vi "event_key_down.vi"(8 "error in":errorcluster, 9 "reference cluster in":T1, 11 "Char":i16) -> (0 "error out":errorcluster)   [LabVIEW 2016]
uses:
  Type Definitions/reference_cluster.ctl
  Type Definitions/vars_settings.ctl
  Type Definitions/stim_type.ctl
  Type Definitions/backlight_type.ctl
  Type Definitions/vars_runtime.ctl
  Type Definitions/data.ctl
  Type Definitions/notifier_elements_GUI.ctl
  Type Definitions/notifier_elements_DAQ.ctl
  Type Definitions/notifier_elements_write.ctl
  Type Definitions/control_references.ctl
types:
  T1 = typedef "reference_cluster.ctl" = cluster{"Vars":cluster{"General":refnum<notifier>, "Runtime":refnum<notifier>}, "Data":cluster{"Display":refnum<queue>, "Write":refnum<queue>}, "LoopCtrl":cluster{"Display":refnum<notifier>, "DAQ":refnum<notifier>, "Write":refnum<notifier>[]}, "Controls":T2, "Error Event":refnum<user-event>}
  T2 = typedef "control_references.ctl" = cluster{"Base Directory":refnum<vi>, "Config File":refnum<vi>, "Timing Issues":refnum<vi>, "Quit":refnum<vi>, "Animal ID":refnum<vi>[], "Session ID":refnum<vi>[], "Active":refnum<vi>[], "Temperature Charts":refnum<vi>[], "Lick Charts":refnum<vi>[], "Bool Displays":refnum<vi>[], "Stimulus Timing":refnum<vi>[], "Stimulus Stats":refnum<vi>[], "Catch Stats":refnum<vi>[], "Recording Status":refnum<vi>[]}
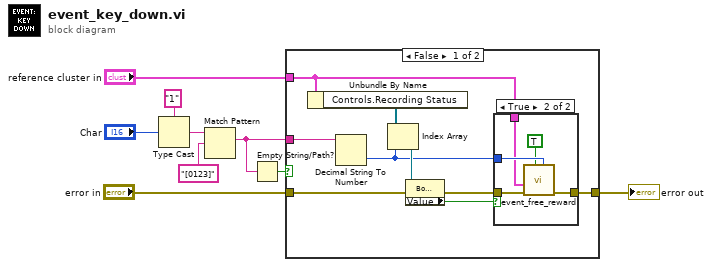
[diagram p0: block diagram]
diagram:
  n1 = Type Cast(type="1" ("String"), x="Char") -> (*(type *) &x=w4:string)
  n2 = Match Pattern(string=w4, regular expression="[0123]") -> (match substring=w2:string)  [unwired: 1 in, 3 out]
  n3 = Empty String/Path?(string/path=w2) -> (empty?=w7:bool)
  n4 = case shown="False" w7 {
    tunnel: w2 -> [w18 _]
    tunnel: "error in" -> [w15 w25]
    tunnel: "reference cluster in" -> [w11 _]
    tunnel: [w10 w25] -> w5
    frame False {
      n5 = Unbundle By Name(w11) -> ("Controls.Recording Status"=w17:refnum<vi>[])
      n6 = Decimal String To Number(string=w18) -> (number=w14:i32)  [unwired: 2 in, 1 out]
      n7 = Index Array(array=w17, index=w14) -> (element=w16:refnum<vi>)
      n8 = property class="Bool (strict)"(reference=w16, error in=w15) -> (error out=w12:errorcluster, "Value"=w13:bool)  [unwired: 1 out]
      n9 = case shown="True" w13 {
        tunnel: w14 -> [_ w23]
        tunnel: w12 -> [w19 w24]
        tunnel: [w19 w22] -> w10
        tunnel: w11 -> [_ w21]
        frame False {
        }
        frame True {
          n10 = call "event_free_reward.vi"("Setup ID"=w23, "New Value"=TRUE, "error in"=w24, "reference cluster in"=w21) -> ("error out"=w22:errorcluster)  [unwired: 7 in]
        }
      }
    }
    frame True {
    }
  }
  "error out" <- w5
